vi "test_LoadFrameEditorFile_v1.vi"(11 "BIN file path":path=path "/home/lvuser/T2_TxRxMon_HARDWARE_board0_v1.bin") -> (0 "error out":errorcluster, 3 "data":T1[](array[typedef]) {"value"."Data" format="%.0x"; "value"."HeaderInfo"."NetSelect" items=["FDX_TX_FRAME_DLY_A"=0, "FDX_TX_FRAME_DLY_B"=1, "FDX_TX_FRAME_BOTH "=3, "FDX_TX_FRAME_ONLY_A"=4, "FDX_TX_FRAME_ONLY_B "=5]; "value"."HeaderInfo"."FrameStartMode" items=["FDX_TX_FRAME_START_IFG", "FDX_TX_FRAME_START_PGWT", "FDX_TX_FRAME_START_TRG"]; "value"."HeaderInfo"."PhysErrorInjection" items=["FDX_TX_FRAME_ERR_OFF"=0, "FDX_TX_FRAME_ERR_CRC"=1, "FDX_TX_FRAME_ERR_ALI"=2, "FDX_TX_FRAME_ERR_PRE"=4, "FDX_TX_FRAME_ERR_PHY"=8]; "value"."HeaderInfo"."SequenceNumberInit" items=["FDX_TX_FRAME_SEQ_INIT_AUTO"=65535]; "value"."HeaderInfo"."SequenceNumberOffset" items=["FDX_TX_FRAME_SEQ_OFFS_AUTO "=65535]; "value"."HeaderInfo"."PayloadGenerationMode" items=["FDX_TX_FRAME_PGM_USER"=0, "FDX_TX_FRAME_PGM_IP_PART"=1, "FDX_TX_FRAME_PGM_IP_FULL"=2, "FDX_TX_FRAME_PGM_IP_PART_TT"=10, "FDX_TX_FRAME_PGM_IP_FULL_TT"=20]; "value"."HeaderInfo"."PayloadBufferMode" items=["FDX_TX_FRAME_PBM_STD", "FDX_TX_FRAME_PBM_MAC", "FDX_TX_FRAME_PBM_UDP"]})   [LabVIEW 2020]
uses:
  Program Files/National Instruments/LabVIEW 2024/instr.lib/AIM GmbH/_AIM 664/helpers/EthFrameManagement/EthFrameManagement.lvlib
  Program Files/National Instruments/LabVIEW 2024/instr.lib/AIM GmbH/_AIM 664/_controls/queue_header_generic.ctl
  Program Files/National Instruments/LabVIEW 2024/instr.lib/AIM GmbH/_AIM 664/AIM664LV.lvlib
  Frame Configuration/controls/frame_record_type.ctl
  Frame Configuration/controls/frame_file_entry.ctl
  Program Files/National Instruments/LabVIEW 2024/instr.lib/AIM GmbH/_AIM 664/helpers/EthFrameManagement/controls/ehternetFrame_type.ctl
  Program Files/National Instruments/LabVIEW 2024/instr.lib/AIM GmbH/_AIM 664/helpers/EthFrameManagement/controls/IPFrame_type.ctl
  Program Files/National Instruments/LabVIEW 2024/instr.lib/AIM GmbH/_AIM 664/helpers/EthFrameManagement/controls/UDPFrame_type.ctl
panel:
  out "Size - Frame":i32=22
  in  "frame index":i32
  out "dst ip":string="224.224.0.60"
  out "src ip":string="10.1.33.1"
  out "Size - payload and CRC":i32=22
  out "UDP header":T4={"Source Port"=1, "Dest Port"=1, "Lenght"=25, "Checksum"=0}
  out "IP header":T5={"Version"=4, "IHL"=5, "ToS"=0, "Length"=45, "ID"=0, "CtlFlags"=2, "FragOffset"=0, "TTL"=1, "Protocol"=17, "Checksum"=28066, "Source IP"=167846145, "Dest IP"=3772776508} {"CtlFlags" format="%.0b"; "Dest IP" format="%.0x"; "Source IP" format="%.0x"; "Checksum" format="%.0x"; "TTL" format="%.0x"; "FragOffset" format="%.0x"; "ID" format="%.0x"; "Length" format="%.0x"; "ToS" format="%.0x"; "IHL" format="%.0x"; "Version" format="%.0x"}
  out "UDP Header Only":u8[](array[numeric])=[0, 1, 0, 1, 0, 25, 0, 0]
  out "IP Header Only":u8[](array[numeric])=[69, 0, 0, 45, 0, 0, 64, 0, 1, 17, 109, 162, 10, 1, 33, 1, 224, 224, 0, 60] format="%.0x"
  out "Ethernet header":T6={"Dest MAC"=[3, 0, 0, 0, 0, 60], "Src MAC"=[2, 0, 0, 1, 33, 32], "EtherType"=2048} {"EtherType" format="%04x"; "Src MAC" format="%02x"; "Dest MAC" format="%.0b"}
  out "MAC Header Only":u8[](array[numeric])=[3, 0, 0, 0, 0, 60, 2, 0, 0, 1, 33, 32, 8, 0] format="%.0x"
  out "payload":u8[](array[numeric]) format="%.0x"
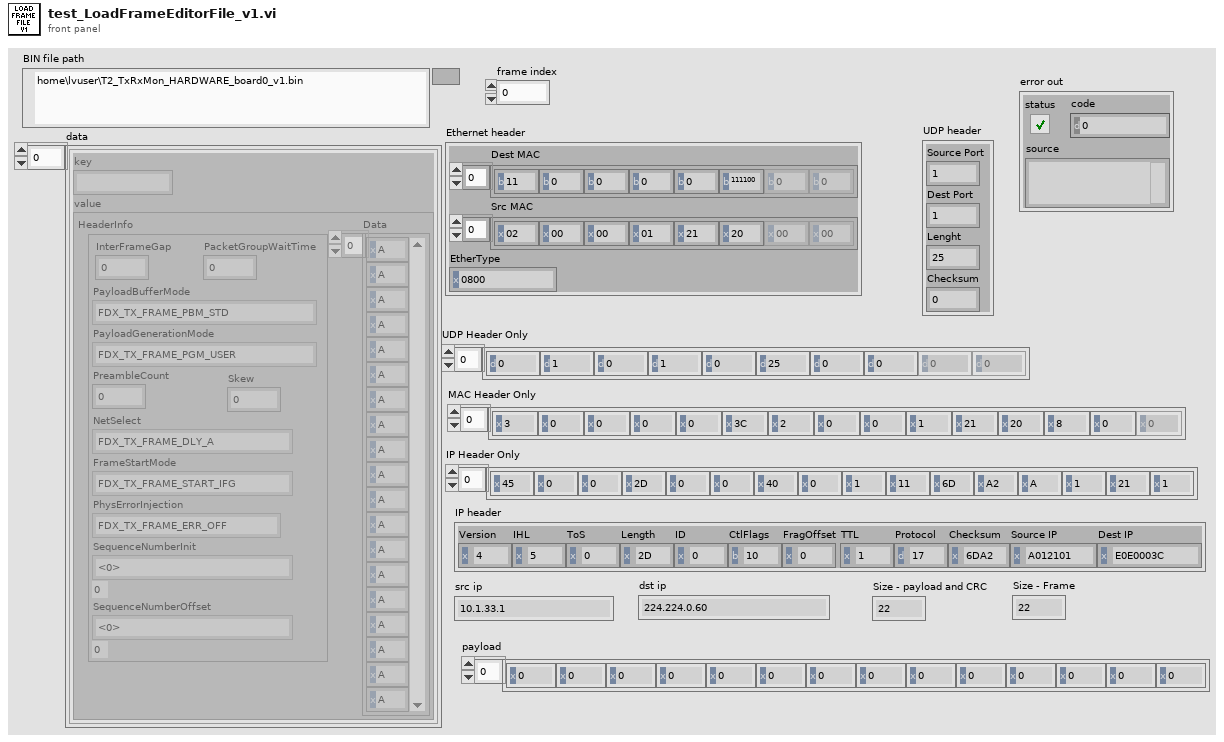
[diagram p1: front panel]
types:
  T1 = typedef "frame_file_entry.ctl" = cluster{"key":string, "value":T2}
  T2 = typedef "frame_record_type.ctl" = cluster{"HeaderInfo":T3, "Data":u8[]}
  T3 = typedef "AIM664LV.lvlib/queue_header_generic.ctl" = cluster{"InterFrameGap":u32, "PacketGroupWaitTime":u32, "PayloadBufferMode":u8, "PayloadGenerationMode":u8, "PreambleCount":u8, "Skew":u32, "NetSelect":u8, "FrameStartMode":u8, "PhysErrorInjection":u32, "SequenceNumberInit":u16, "SequenceNumberOffset":u16}
  T4 = typedef "EthFrameManagement.lvlib/UDPFrame_type.ctl" = cluster{"Source Port":u16, "Dest Port":u16, "Lenght":u16, "Checksum":u16}
  T5 = typedef "EthFrameManagement.lvlib/IPFrame_type.ctl" = cluster{"Version":u8, "IHL":u8, "ToS":u8, "Length":u16, "ID":u16, "CtlFlags":u8, "FragOffset":u16, "TTL":u8, "Protocol":u8, "Checksum":u16, "Source IP":u32, "Dest IP":u32}
  T6 = typedef "EthFrameManagement.lvlib/ehternetFrame_type.ctl" = cluster{"Dest MAC":u8[], "Src MAC":u8[], "EtherType":u16}
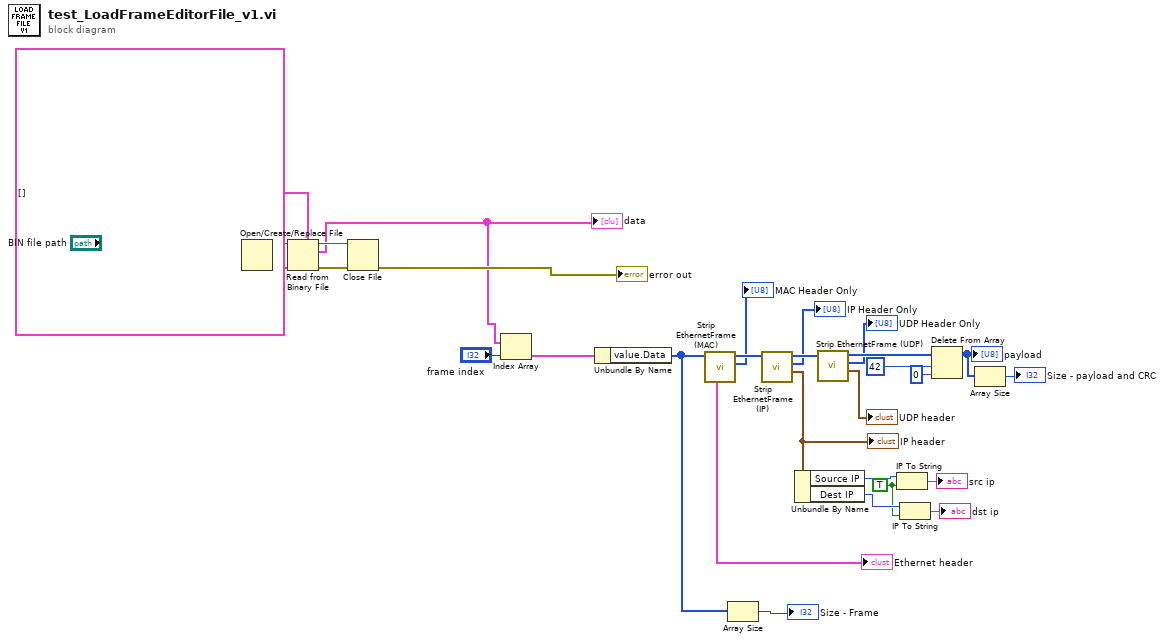
[diagram p0: block diagram]
diagram:
  w8 = TRUE ("dot notation? (F)")
  n1 = Open/Create/Replace File(file path (use dialog)="BIN file path") -> (refnum out=w28:refnum<file>, error out=w27:errorcluster)  [unwired: 5 in, 1 out]
  n2 = Read from Binary File(5:T1[] [] ("Array"), 8:w27, 11:w28) -> (0:w29:errorcluster, 2:w3:T1[], 3:w30:refnum<file>)  [unwired: 3 in, 1 out]
  "data" <- w3
  n3 = Close File(refnum=w30, error in=w29) -> (error out=→"error out":errorcluster)  [unwired: 1 out]
  n4 = Index Array(array=w3, index="frame index") -> (element=w24:T1)
  n5 = Unbundle By Name(w24) -> ("value.Data"=w2:u8[])
  n6 = call "Strip EthernetFrame (MAC).vi"("Ethernet Frame In"=w2) -> ("Ethernet header"=→"Ethernet header":T6, "MAC Header Only"=→"MAC Header Only":u8[], "Ethernet Frame Out"=w23:u8[])  [unwired: 7 in, 1 out]
  n7 = Array Size(array=w2) -> (size(s)=→"Size - Frame":i32)
  n8 = call "Strip EthernetFrame (IP).vi"("Frame In"=w23) -> ("IP header"=w11:T5, "IP Header Only"=→"IP Header Only":u8[], "Frame Out"=w22:u8[])  [unwired: 7 in, 1 out]
  "IP header" <- w11
  n9 = Unbundle By Name(w11) -> ("Source IP"=w10:u32, "Dest IP"=w9:u32)
  n10 = call "Strip EthernetFrame (UDP).vi"("Ethernet Frame In"=w22) -> ("UDP header"=→"UDP header":T4, "UDP Header Only"=→"UDP Header Only":u8[], "Ethernet Frame Out"=w21:u8[])  [unwired: 7 in, 1 out]
  n11 = IP To String(1:w8, 2:w10) -> (0:→"src ip":string)
  n12 = IP To String(1:w8, 2:w9) -> (0:→"dst ip":string)
  n13 = Delete From Array(array=w21, length=42 ("index"), index=0) -> (array with subset deleted=w13:u8[])  [unwired: 1 out]
  "payload" <- w13
  n14 = Array Size(array=w13) -> (size(s)=→"Size - payload and CRC":i32)
